vi "fg_event_auth.vi"(8 "error in (no error)":errorcluster) -> (0 "error out":errorcluster, 3 "auth":refnum<user-event>)   [LabVIEW 2015, in "lv-dropbox.lvlib" / "examples.lvlib"]
uses:
  examples.lvlib
  _controls/authorization_response.ctl
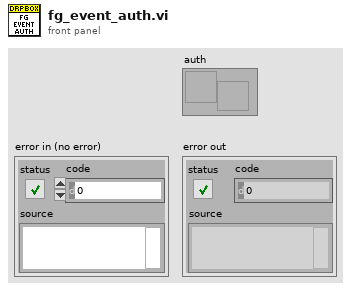
[diagram p1: front panel]
types:
  T1 = typedef "lv-dropbox.lvlib/examples.lvlib/authorization_response.ctl" = cluster{"code":string, "state":string}
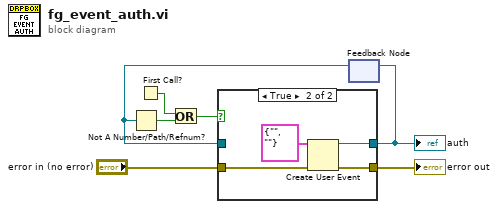
[diagram p0: block diagram]
diagram:
  n1 = First Call?() -> (First Call?: T/F=w1:bool)
  n2 = feedback #1() -> (w4:refnum<user-event>)  [unwired: 1 in]
  n3 = Not A Number/Path/Refnum?(number/path/refnum=w4) -> (NaN/Path/Refnum?=w3:bool)
  n4 = Or(x=w1, y=w3) -> (x .or. y?=w2:bool)
  n5 = case shown="True" w2 {
    tunnel: "error in (no error)" -> [w8 w13]
    tunnel: [w8 w12] -> w6
    tunnel: [w9 w11] -> w5
    tunnel: w4 -> [w9 _]
    frame False {
    }
    frame True {
      n6 = Create User Event(user event datatype=T1 {"code"="", "state"=""} ("auth"), error in=w13) -> (user event=w11:refnum<user-event>, error out=w12:errorcluster)
    }
  }
  "error out" <- w6
  "auth" <- w5
  n7 = feedback-in #1(w5) -> ()
